vi "Lvi Read U32Data Pt.vi"(8 "error in (no error)":errorcluster, 10 "timeout":dbl, 11 "TaskRef":i32) -> (0 "error out":errorcluster, 1 "function return":i32, 2 "DataBuf":u32, 3 "TaskRef out":i32)   [LabVIEW 2022 SP3, in "DtLvLink.lvlib"]
doc: "Calls directly into the entry points of the DLL of the Data Acq SDK to return a data point from the specified task as an unsigned 32-bit integer."
uses:
  DtLvLink.lvlib
  <userlib>/LV-Link3/DtLvLink_64.dll
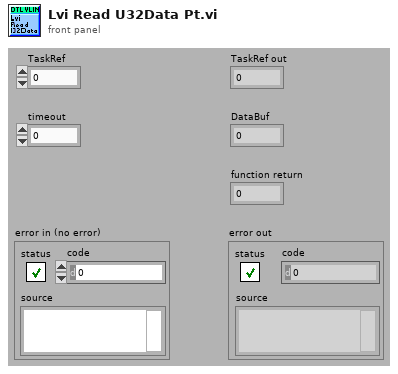
[diagram p1: front panel]
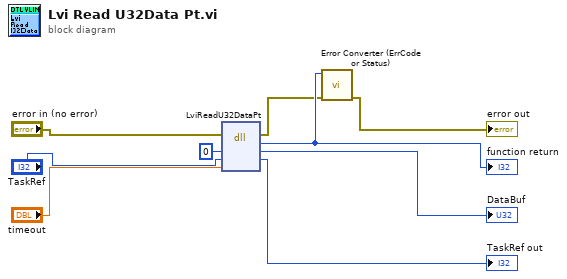
[diagram p0: block diagram]
diagram:
  n1 = dll-call lib="C:/Program Files/National Instruments/LabVIEW 2022/user.lib/LV-Link3/DtLvLink_64.*" fn="LviReadU32DataPt"(error in="error in (no error)", "DataBuf"=u32 0, "TaskRef"="TaskRef", "timeout"="timeout") -> (error out=w2:errorcluster, "return type"=w9:i32, "DataBuf"=→"DataBuf":u32, "TaskRef"=→"TaskRef out":i32)  [unwired: 3 in, 1 out]
  "function return" <- w9
  n2 = call "Error Converter (ErrCode or Status).vi"("error in (no error)"=w2, "error code"=w9) -> ("error out"=→"error out":errorcluster)  [unwired: 9 in]
